vi "Table Pick Row Border.vi"(6 "Data Row Back Ground color":T9={"color"=16777225, "at each"=0.0}, 7 "Row borders from":T8, 8 "Title Row Cells":T6={"Cell Cluster"={"Font Ref"=refnum, "Leading"=18.0, "Horizontal Aligment"=enum."JUSTIFY", "Vertical Alignment"=enum."BOTTOM"}, "PdfPCell [ ]"=[]}, 9 "Datas Row Cells [ ]":T1, 10 "i":i32, 11 "N":i32) -> (1 "Row Borders":T7={"Row"={"#"=0, "to #"=0}, "Cell Cluster"={"Font Ref"=refnum, "Leading"=18.0, "Horizontal Aligment"=enum."JUSTIFY", "Vertical Alignment"=enum."BOTTOM"}, "PdfPCell [ ]"=[]}, 3 "Background Color":u32(colorbox))   [LabVIEW 2012]
doc: "Version 1.0\nDeveloped by Jean-Marc Simard\nCopyright © 2010, Exaprom Inc.\nAll rights reserved.\nLicense: BSD"
uses:
  Controls/Row Back Ground color Datas.ctl
  Controls/Row borders from.ctl
  Controls/Cell Cluster.ctl
  C:/Users/MaxCorp/Documents/TopPerm - Base/DLL/itextsharp.dll
  DLL/itextsharp.dll
  Controls/Font size.ctl
  Controls/Texte alignement.ctl
  Controls/Cell Vertical alignment.ctl
  Controls/Title Cells with refnum.ctl
  Controls/Row PdfPCell [ ] Datas.ctl
panel:
  out "x-y":u32
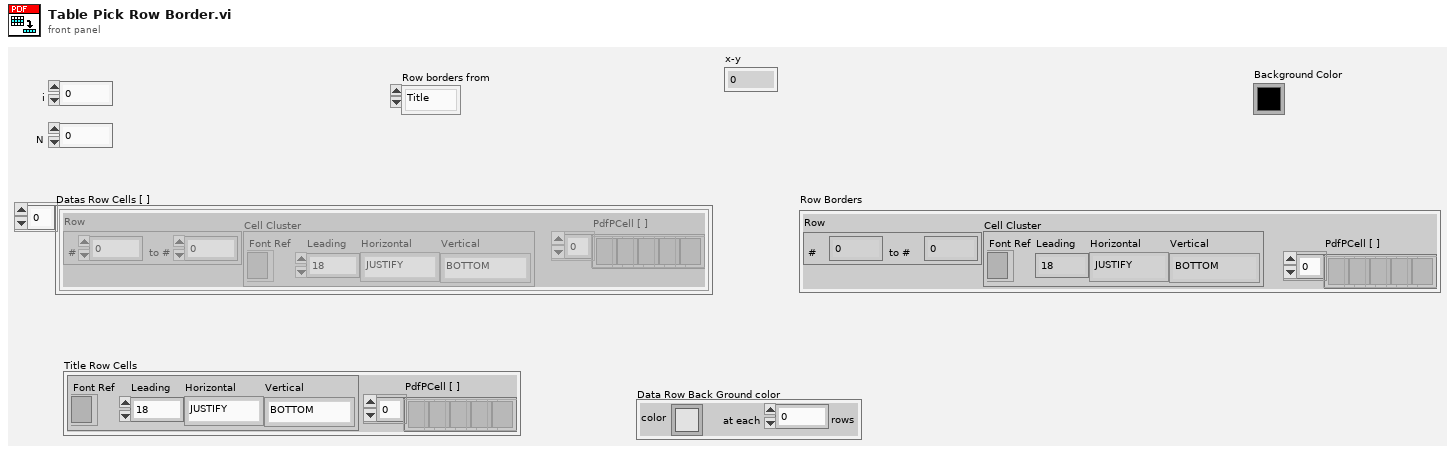
[diagram p1: front panel]
types:
  T1 = typedef "Row PdfPCell [ ] Datas.ctl" = cluster{"Row":cluster{"#":i16, "to #":i16}, "Cell Cluster":T2, "PdfPCell [ ]":refnum<k24>[]}[]
  T2 = typedef "Cell Cluster.ctl" = cluster{"Font Ref":refnum<k24>, "Leading":T3, "Horizontal Aligment":T4, "Vertical Alignment":T5}
  T3 = typedef "Font size.ctl" = sgl
  T4 = typedef "Texte alignement.ctl" = enum16{"Select", "CENTER", "JUSTIFY", "LEFT", "RIGHT"}
  T5 = typedef "Cell Vertical alignment.ctl" = enum16{"TOP", "MIDDLE", "BOTTOM"}
  T6 = typedef "Title Cells with refnum.ctl" = cluster{"Cell Cluster":T2, "PdfPCell [ ]":refnum<k24>[]}
  T7 = cluster{"Row":cluster{"#":i16, "to #":i16}, "Cell Cluster":T2, "PdfPCell [ ]":refnum<k24>[]}
  T8 = typedef "Row borders from.ctl" = enum16{"Title", "Datas"}
  T9 = typedef "Row Back Ground color Datas.ctl" = cluster{"color":u32, "at each":dbl}
  T10 = cluster{"Row":cluster{"#":i16, "to #":i16}, "Cell Cluster":T2, "PdfPCell [ ]":refnum<k24>[]}[]
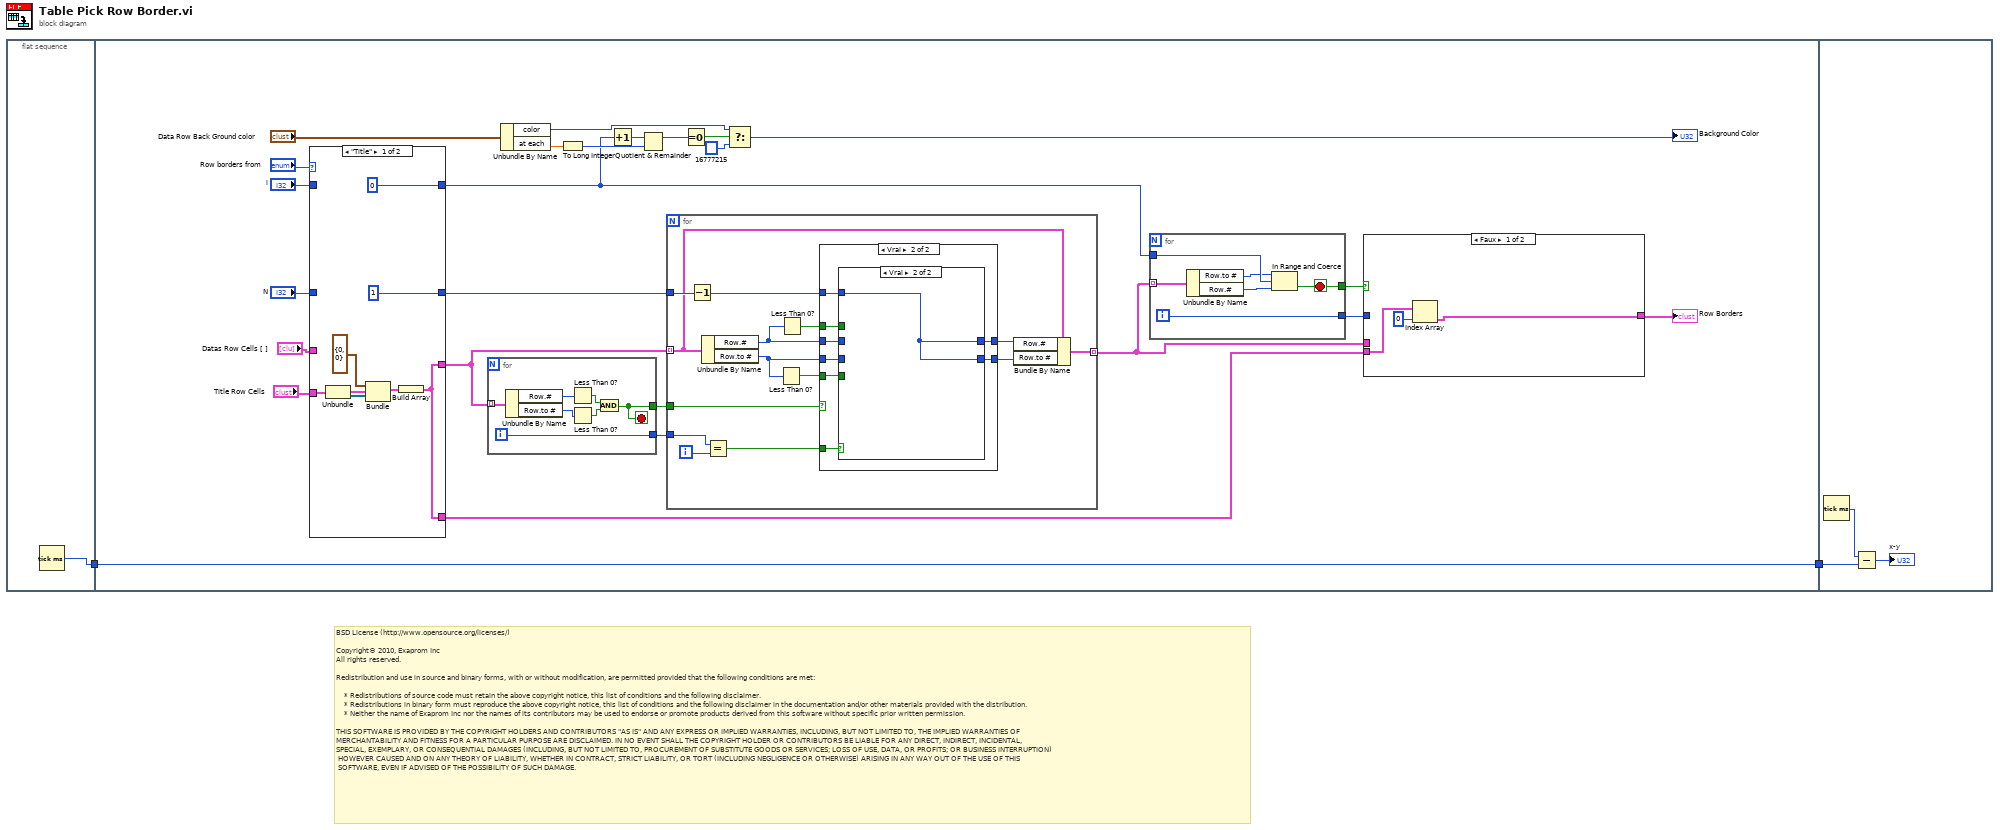
[diagram p0: block diagram]
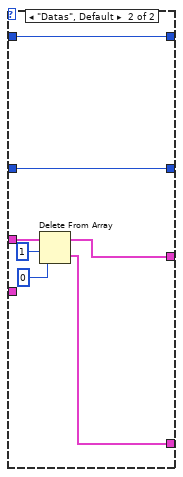
[diagram p2: hidden frame]
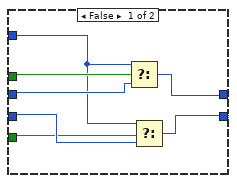
[diagram p3: hidden frame]
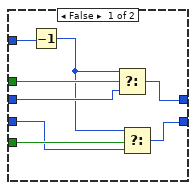
[diagram p4: hidden frame]
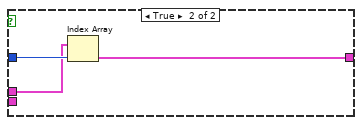
[diagram p5: hidden frame]
diagram:
  # "BSD License (http://www.opensource.org/licenses/)\n\nCopyright© 2010, Exaprom Inc\nAll rights reserved.\n\nRedistribution and use in source and binary forms, with or without modification, are permitted provided that the following conditions are met:\n\n    * Redistributions of source code must retain the above copyright notice, this list of conditions and the following disclaimer.\n    * Redistributions in binary form must reproduce the above copyright notice, this list of conditions and the following disclaimer in the documentation and/or other materials provided with the distribution.\n    * Neither the name of Exaprom Inc nor the names of its contributors may be used to endorse or promote products derived from this software without specific prior written permission.\n\nTHIS SOFTWARE IS PROVIDED BY THE COPYRIGHT HOLDERS AND CONTRIBUTORS \"AS IS\" AND ANY EXPRESS OR IMPLIED WARRANTIES, INCLUDING, BUT NOT LIMITED TO, THE IMPLIED WARRANTIES OF \nMERCHANTABILITY AND FITNESS FOR A PARTICULAR PURPOSE ARE DISCLAIMED. IN NO EVENT SHALL THE COPYRIGHT HOLDER OR CONTRIBUTORS BE LIABLE FOR ANY DIRECT, INDIRECT, INCIDENTAL,\nSPECIAL, EXEMPLARY, OR CONSEQUENTIAL DAMAGES (INCLUDING, BUT NOT LIMITED TO, PROCUREMENT OF SUBSTITUTE GOODS OR SERVICES; LOSS OF USE, DATA, OR PROFITS; OR BUSINESS INTERRUPTION)\n HOWEVER CAUSED AND ON ANY THEORY OF LIABILITY, WHETHER IN CONTRACT, STRICT LIABILITY, OR TORT (INCLUDING NEGLIGENCE OR OTHERWISE) ARISING IN ANY WAY OUT OF THE USE OF THIS\n SOFTWARE, EVEN IF ADVISED OF THE POSSIBILITY OF SUCH DAMAGE."
  n1 = flat-sequence {
    tunnel: [w3] -> w1
    tunnel: [w4] -> w2
    tunnel: w1 -> [w4]
    tunnel: w2 -> [w101]
    frame #0 {
      n2 = Tick Count (ms)() -> (millisecond timer value=w3:u32)
    }
    frame #1 {
      n3 = case shown="\"Title\"" "Row borders from" {
        tunnel: [0 ("i") w43] -> w14
        tunnel: "i" -> [_ w43]
        tunnel: [1 ("N") w42] -> w12
        tunnel: "N" -> [_ w42]
        tunnel: [w29 w40] -> w10
        tunnel: "Datas Row Cells [ ]" -> [_ w41]
        tunnel: "Title Row Cells" -> [w34 _]
        tunnel: [w29 w37] -> w6
        frame "Title" {
          n4 = Unbundle(w34) -> ("Cell Cluster"=w33:T2, "PdfPCell [ ]"=w31:refnum<k24>[])
          n5 = Bundle("Row"=cluster{"#":i16, "to #":i16} {"#"=0, "to #"=0}, "Cell Cluster"=w33, "PdfPCell [ ]"=w31) -> (w30:T7)  [unwired: 1 out]
          n6 = Build Array(w30) -> (w29:T10)
        }
        frame "Datas", Default {
          n7 = Delete From Array(array=w41, length=1, index=0) -> (deleted portion=w37:T1, array with subset deleted=w40:T1)
        }
      }
      n8 = for {
        tunnel: w10 -> [w88] mode=indexing
        tunnel: [w83] -> w26
        tunnel: [w82] -> w25
        i -> [w82]
        stop <- w83 stop-if-true
        n9 = Unbundle By Name(w88) -> ("Row.#"=w87:i16, "Row.to #"=w86:i16)
        n10 = Less Than 0?(x=w87) -> (x < 0?=w84:bool)
        n11 = Less Than 0?(x=w86) -> (x < 0?=w85:bool)
        n12 = And(x=w84, y=w85) -> (x .and. y?=w83:bool)
      }
      n13 = Unbundle By Name("Data Row Back Ground color") -> ("color"=w18:u32, "at each"=w23:dbl)
      n14 = To Long Integer(number=w23) -> (32bit integer=w22:i32)
      n15 = Increment(x=w14) -> (x+1=w21:i32)
      n16 = Quotient & Remainder(x=w21, y=w22) -> (x-y*floor(x/y)=w20:i32)  [unwired: 1 out]
      n17 = for {
        tunnel: w10 -> [w49] mode=indexing
        tunnel: w26 -> [w57]
        tunnel: w25 -> [w55]
        tunnel: w12 -> [w51]
        tunnel: [w44] -> w5 mode=indexing
        i -> [w56]
        n18 = Decrement(x=w51) -> (x-1=w50:i32)
        n19 = Unbundle By Name(w49) -> ("Row.#"=w53:i16, "Row.to #"=w52:i16)
        n20 = Equal?(x=w55, y=w56) -> (x = y?=w54:bool)
        n21 = Less Than 0?(x=w52) -> (x < 0?=w46:bool)
        n22 = Less Than 0?(x=w53) -> (x < 0?=w45:bool)
        n23 = case shown="Vrai" w57 {
          tunnel: w54 -> [_ w72]
          tunnel: w53 -> [w64 w71]
          tunnel: w52 -> [w62 w70]
          tunnel: w50 -> [w58 w69]
          tunnel: [w59 w68] -> w48
          tunnel: [w60 w67] -> w47
          tunnel: w46 -> [w61 w66]
          tunnel: w45 -> [w63 w65]
          frame False {
            n24 = Select(t=w58, s=w63, f=w64) -> (s? t:f=w59:i32)
            n25 = Select(t=w58, s=w61, f=w62) -> (s? t:f=w60:i32)
          }
          frame True {
            n26 = case shown="Vrai" w72 {
              tunnel: w71 -> [w78 _]
              tunnel: w70 -> [w74 _]
              tunnel: [w77 w81] -> w68
              tunnel: [w73 w81] -> w67
              tunnel: w69 -> [w80 w81]
              tunnel: w66 -> [w76 _]
              tunnel: w65 -> [w79 _]
              frame False {
                n27 = Decrement(x=w80) -> (x-1=w75:i32)
                n28 = Select(t=w75, s=w79, f=w78) -> (s? t:f=w77:i32)
                n29 = Select(t=w75, s=w76, f=w74) -> (s? t:f=w73:i32)
              }
              frame True {
              }
            }
          }
        }
        n30 = Bundle By Name(cluster=w49, "Row.#"=w48, "Row.to #"=w47) -> (w44:T7)
      }
      n31 = Equal To 0?(x=w20) -> (x = 0?=w19:bool)
      n32 = Select(t=w18, s=w19, f=u32 16777215 ("Color")) -> (s? t:f=→"Background Color":u32)
      n33 = for {
        tunnel: w5 -> [w100] mode=indexing
        tunnel: w14 -> [w99]
        tunnel: [w98] -> w27
        tunnel: [w96] -> w28
        i -> [w98]
        stop <- w96 stop-if-true
        n34 = Unbundle By Name(w100) -> ("Row.to #"=w95:i16, "Row.#"=w97:i16)
        n35 = In Range and Coerce(upper limit=w95, x=w99, lower limit=w97) -> (In Range?=w96:bool)  [unwired: 1 out]
      }
      n36 = case shown="Faux" w28 {
        tunnel: w27 -> [_ w94]
        tunnel: w6 -> [w91 _]
        tunnel: [w89 w93] -> w7
        tunnel: w5 -> [_ w92]
        frame False {
          n37 = Index Array(array=w91, index=0) -> (element=w89:T7)
        }
        frame True {
          n38 = Index Array(array=w92, index=w94) -> (element=w93:T7)
        }
      }
      "Row Borders" <- w7
    }
    frame #2 {
      n39 = Tick Count (ms)() -> (millisecond timer value=w103:u32)
      n40 = Subtract(x=w103, y=w101) -> (x-y=→"x-y":u32)
    }
  }
